vi "Export Configuration.vi"() -> ()   [LabVIEW 2015]
uses:
  <vilib>/nisyscfg/nisyscfg.lvlib
panel:
  in  "Destination File":path=path "C:/Users/Matt/Desktop/exscalabar.nce"
  in  "Session in":refnum<k21>="exscalabar (192.168.0.73)"
  out "error out":errorcluster
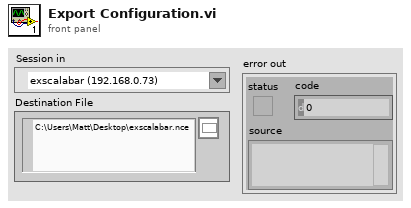
[diagram p1: front panel]
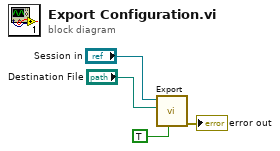
[diagram p0: block diagram]
diagram:
  n1 = call <vilib>:"Export.vi"("Overwrite (F)"=TRUE, "Destination File"="Destination File", "Session in"="Session in") -> ("error out"=→"error out":errorcluster)  [unwired: 7 in, 1 out]
